vi "Konwersja_Num_na_TypUsr.vi"(10 "Zakres No":i32) -> (2 "Typ pomiaru":T1(ring))   [LabVIEW 2014]
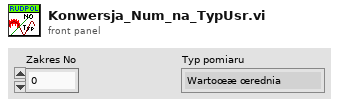
[diagram p1: front panel]
types:
  T1 = enum16{"Wartoœæ œrednia", "Œrednia wyprostowana", "Wartoœæ skuteczna"}
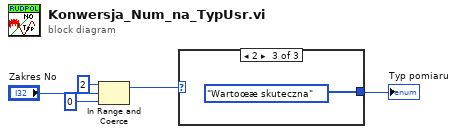
[diagram p0: block diagram]
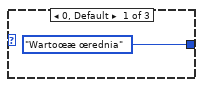
[diagram p2: hidden frame]
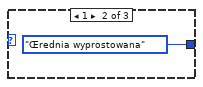
[diagram p3: hidden frame]
diagram:
  n1 = In Range and Coerce(upper limit=2, x="Zakres No", lower limit=0) -> (coerced(x)=w2:i32)  [unwired: 1 out]
  n2 = case shown="2" w2 {
    tunnel: [T1."Wartoœæ œrednia" ("Typ pomiaru 2") T1."Œrednia wyprostowana" ("Typ pomiaru 2") T1."Wartoœæ skuteczna" ("Typ pomiaru 2")] -> w1
    frame 0, Default {
    }
    frame 1 {
    }
    frame 2 {
    }
  }
  "Typ pomiaru" <- w1
